vi "pallet labeling.vi"(0 "info array":dbl[][](array[numeric]), 2 "pallet num":i32, 4 "curv num":i32, 6 "error in (no error)":errorcluster) -> (20 "curv plt color":cluster{u32, u32}, 21 "pallet colour":cluster{u32, u32}, 23 "gratbar statuse":i8, 24 "pallet_sit":i8, 25 "alarm":bool, 26 "Color Box":u32(colorbox), 27 "error out":errorcluster)   [LabVIEW 2019]
panel:
  out "2nd thr":dbl=50.0
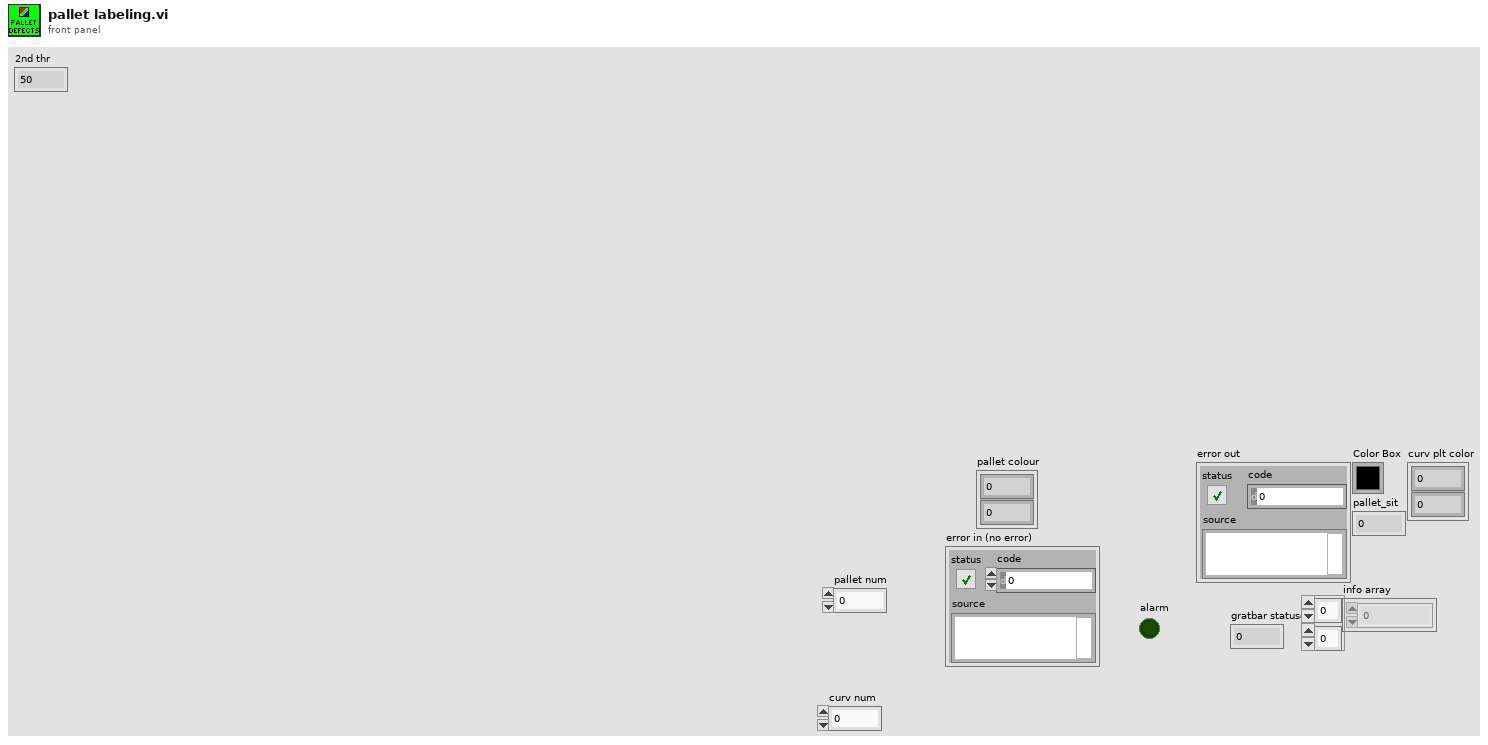
[diagram p1: front panel]
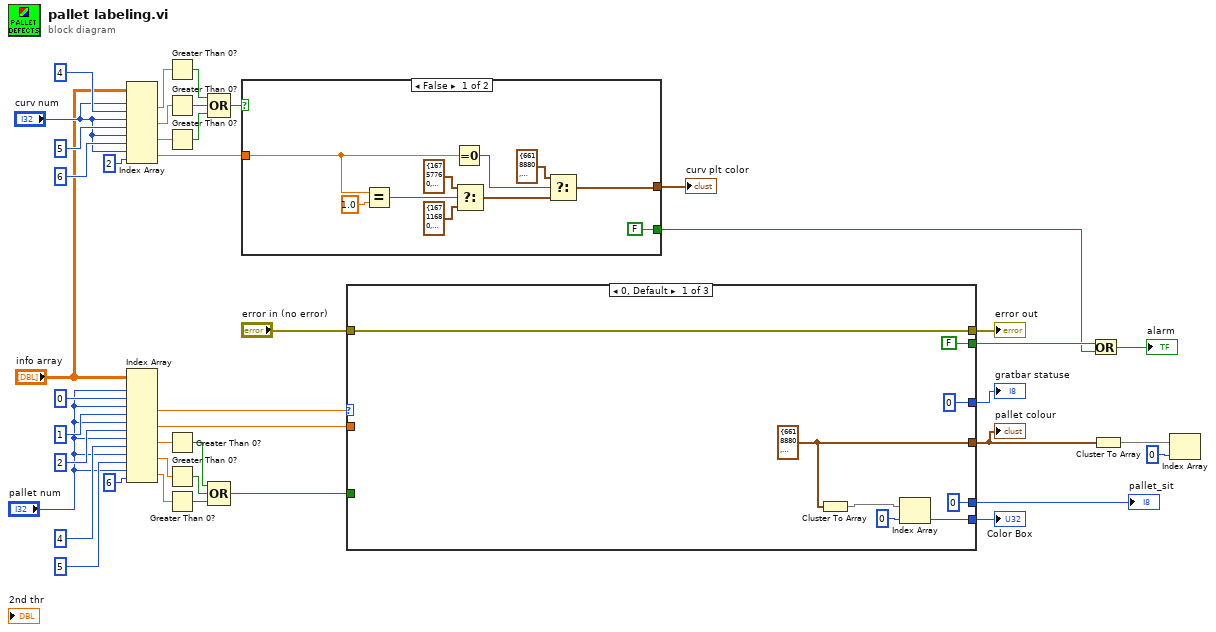
[diagram p0: block diagram]
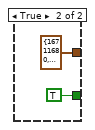
[diagram p2: hidden frame]
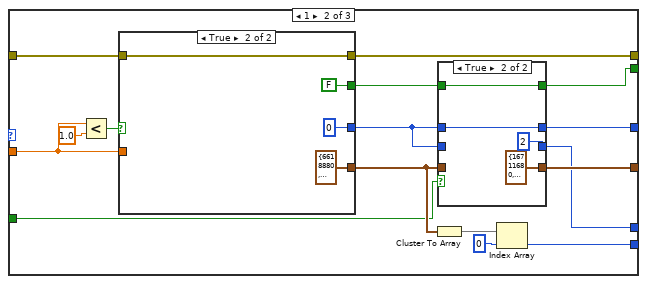
[diagram p3: hidden frame]
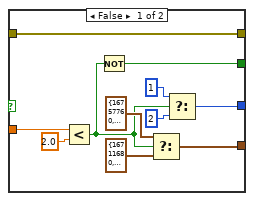
[diagram p5: hidden frame]
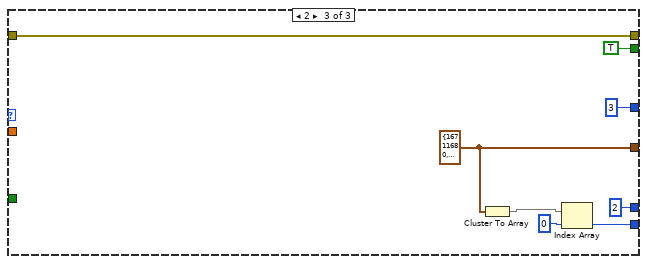
[diagram p6: hidden frame]
diagram:
  n1 = Index Array(array="info array", index (row) #1="curv num", index (col) #1=4 ("disabled index (col)"), index (row) #2="curv num", index (col) #2=5 ("disabled index (col)"), index (row) #3="curv num", index (col) #3=6 ("disabled index (col)"), index (row) #4="curv num", index (col) #4=2 ("disabled index (col)")) -> (element #1=w9:dbl, element #2=w8:dbl, element #3=w7:dbl, element #4=w24:dbl)
  n2 = Index Array(array="info array", index (row) #1="pallet num", index (col) #1=0 ("disabled index (col)"), index (row) #2="pallet num", index (col) #2=1 ("disabled index (col)"), index (row) #3="pallet num", index (col) #3=2 ("disabled index (col)"), index (row) #4="pallet num", index (col) #4=4 ("index (col)"), index (row) #5="pallet num", index (col) #5=5 ("index (col)"), index (row) #6="pallet num", index (col) #6=6 ("index (col)")) -> (element #2=w23:dbl, element #3=w22:dbl, element #4=w17:dbl, element #5=w16:dbl, element #6=w15:dbl)  [unwired: 1 out]
  n3 = Greater Than 0?(x=w9) -> (x > 0?=w32:bool)
  n4 = Greater Than 0?(x=w8) -> (x > 0?=w33:bool)
  n5 = Greater Than 0?(x=w7) -> (x > 0?=w34:bool)
  n6 = Greater Than 0?(x=w17) -> (x > 0?=w14:bool)
  n7 = Greater Than 0?(x=w16) -> (x > 0?=w13:bool)
  n8 = Greater Than 0?(x=w15) -> (x > 0?=w12:bool)
  n9 = Compound Arithmetic op=OR(w32, w33, w34) -> (w26:bool)
  n10 = Compound Arithmetic op=OR(w14, w13, w12) -> (w11:bool)
  n11 = case shown="False" w26 {
    tunnel: [w45 cluster{u32, u32} {16711680, 16711680} ("new element/subarray")] -> w25
    tunnel: w24 -> [w44 _]
    tunnel: [FALSE TRUE] -> w4
    frame False {
      n12 = Equal?(x=w44, y=1.0) -> (x = y?=w49:bool)
      n13 = Equal To 0?(x=w44) -> (x = 0?=w52:bool)
      n14 = Select(t=cluster{u32, u32} {16757760, 16763714} ("new element/subarray"), s=w49, f=cluster{u32, u32} {16711680, 16711680} ("new element/subarray")) -> (s? t:f=w46:cluster{u32, u32})
      n15 = Select(t=cluster{u32, u32} {6618880, 6618880} ("new element/subarray"), s=w52, f=w46) -> (s? t:f=w45:cluster{u32, u32})
    }
    frame True {
    }
  }
  "curv plt color" <- w25
  n16 = case shown="0, Default" w23 {
    tunnel: [w57 w75 w104] -> w40
    tunnel: "error in (no error)" -> [w62 w77 w109]
    tunnel: [w62 w76 w109] -> w41
    tunnel: [FALSE ("Boolean") w73 TRUE ("Boolean")] -> w5
    tunnel: [i8 0 ("gratbar statuse") w74 i8 3 ("gratbar statuse")] -> w2
    tunnel: w22 -> [_ w67 _]
    tunnel: w11 -> [_ w66 _]
    tunnel: [w56 w65 w103] -> w6
    tunnel: [i8 0 ("gratbar statuse") w63 i8 2 ("gratbar statuse")] -> w1
    frame 0, Default {
      w57 = cluster{u32, u32} {6618880, 6618880} ("new element/subarray")
      n17 = Cluster To Array(cluster=w57) -> (array=w59:u32[])
      n18 = Index Array(array=w59, index=0) -> (element=w56:u32)
    }
    frame 1 {
      n19 = Less?(x=w67, y=1.0) -> (x < y?=w78:bool)
      n20 = case shown="True" w78 {
        tunnel: [w95 cluster{u32, u32} {6618880, 6618880} ("new element/subarray")] -> w69
        tunnel: w77 -> [w94 w100]
        tunnel: [w94 w100] -> w76
        tunnel: [w89 FALSE ("Boolean")] -> w72
        tunnel: [w91 i8 0 ("gratbar statuse")] -> w64
        tunnel: w67 -> [w88 _]
        frame False {
          n21 = Less?(x=w88, y=2.0) -> (x < y?=w90:bool)
          n22 = Not(x=w90) -> (.not. x?=w89:bool)
          n23 = Select(t=cluster{u32, u32} {16757760, 16763714} ("new element/subarray"), s=w90, f=cluster{u32, u32} {16711680, 16711680} ("new element/subarray")) -> (s? t:f=w95:cluster{u32, u32})
          n24 = Select(t=i8 1, s=w90, f=i8 2) -> (s? t:f=w91:i8)
        }
        frame True {
        }
      }
      n25 = Cluster To Array(cluster=w69) -> (array=w70:u32[])
      n26 = case shown="True" w66 {
        tunnel: [w82 cluster{u32, u32} {16711680, 16711680} ("new element/subarray")] -> w75
        tunnel: w69 -> [w82 _]
        tunnel: [w81 w85] -> w74
        tunnel: w64 -> [w81 w85]
        tunnel: [w80 w84] -> w73
        tunnel: w72 -> [w80 w84]
        tunnel: w64 -> [w79 _]
        tunnel: [w79 i8 2 ("gratbar statuse")] -> w63
        frame False {
        }
        frame True {
        }
      }
      n27 = Index Array(array=w70, index=0) -> (element=w65:u32)
    }
    frame 2 {
      w104 = cluster{u32, u32} {16711680, 16711680} ("new element/subarray")
      n28 = Cluster To Array(cluster=w104) -> (array=w105:u32[])
      n29 = Index Array(array=w105, index=0) -> (element=w103:u32)
    }
  }
  "pallet colour" <- w40
  "error out" <- w41
  "gratbar statuse" <- w2
  "pallet_sit" <- w1
  "Color Box" <- w6
  n30 = Or(x=w5, y=w4) -> (x .or. y?=→"alarm":bool)
  n31 = Cluster To Array(cluster=w40) -> (array=w39:u32[])
  n32 = Index Array(array=w39, index=0) -> ()  [unwired: 1 out]
